vi "get_Jog.vi"(0 "路径":path, 2 "坐标转换":dbl[](array[numeric]), 3 "初始化？":bool, 4 "error in (no error)":errorcluster caption="错误输入（无错误）") -> (1 "上次限位":dbl, 5 "上一次位置":i32[](array[numeric]), 6 "File Out":path, 7 "坐标位置":dbl[][](array[numeric])=[[0.0, 1000.0, 2000.0, 3000.0], [0.0, 1000.0, 2000.0, 3000.0], [0.0, 1000.0, 2000.0, 3000.0], [0.0, 1000.0, 2000.0, 3000.0], [0.0, 1000.0, 2000.0, 3000.0]], 8 "当前位置":string[](array[string]), 9 "error out":errorcluster, 10 "工位名称":cluster{"String":string, "数值":i32}[](array[cluster]))   [LabVIEW 2018]
uses:
  <vilib>/Utility/file.llb/Write Delimited Spreadsheet (DBL).vi
  <vilib>/Utility/file.llb/Write Delimited Spreadsheet (string).vi
  <vilib>/Utility/file.llb/Read Delimited Spreadsheet (string).vi
panel:
  in  "table 4":string
  in  "table 3":string
  in  "table 2":string
  in  "table1":string
  in  "退出":bool caption="按钮"
  in  "确定":bool caption="按钮"
  in  "位置":dbl[][](array[numeric])=[[0.0, 100.0, 200.0, 300.0], [0.0, 100.0, 200.0, 300.0], [0.0, 100.0, 200.0, 300.0], [0.0, 1000.0, 2000.0, 3000.0], [0.0, 1000.0, 2000.0, 3000.0], [0.0, 1000.0, 2000.0, 3000.0]] min=0.0
  # "大平台X mm"
  # "大平台Y mm"
  # "大平台Z mm"
  # "小平台X mm"
  # "大平台Y mm"
  # "小平台Z mm"
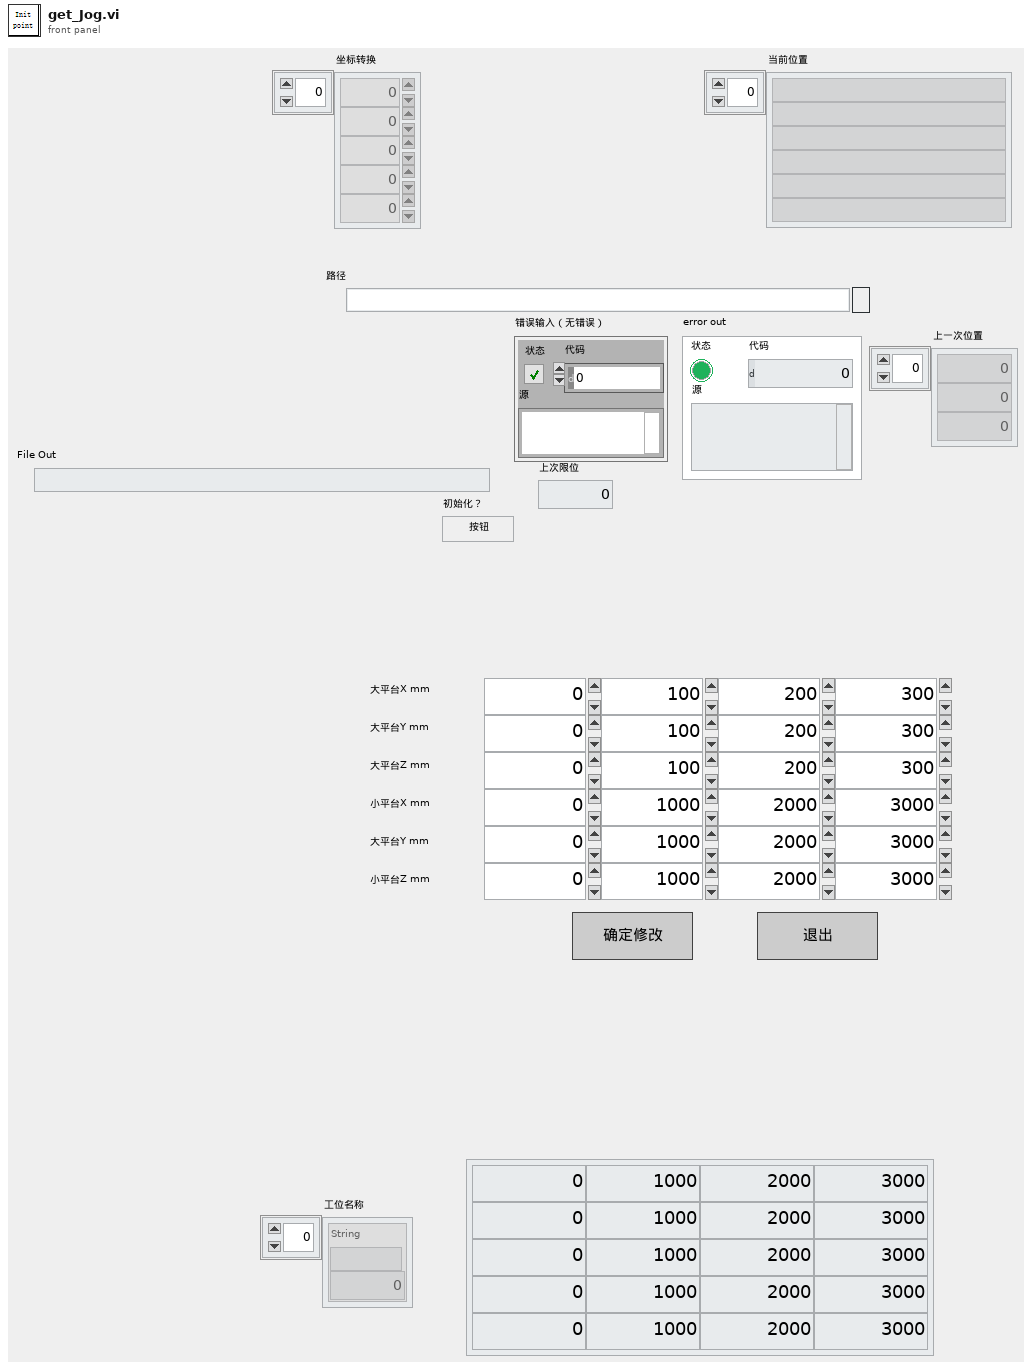
[diagram p1: front panel]
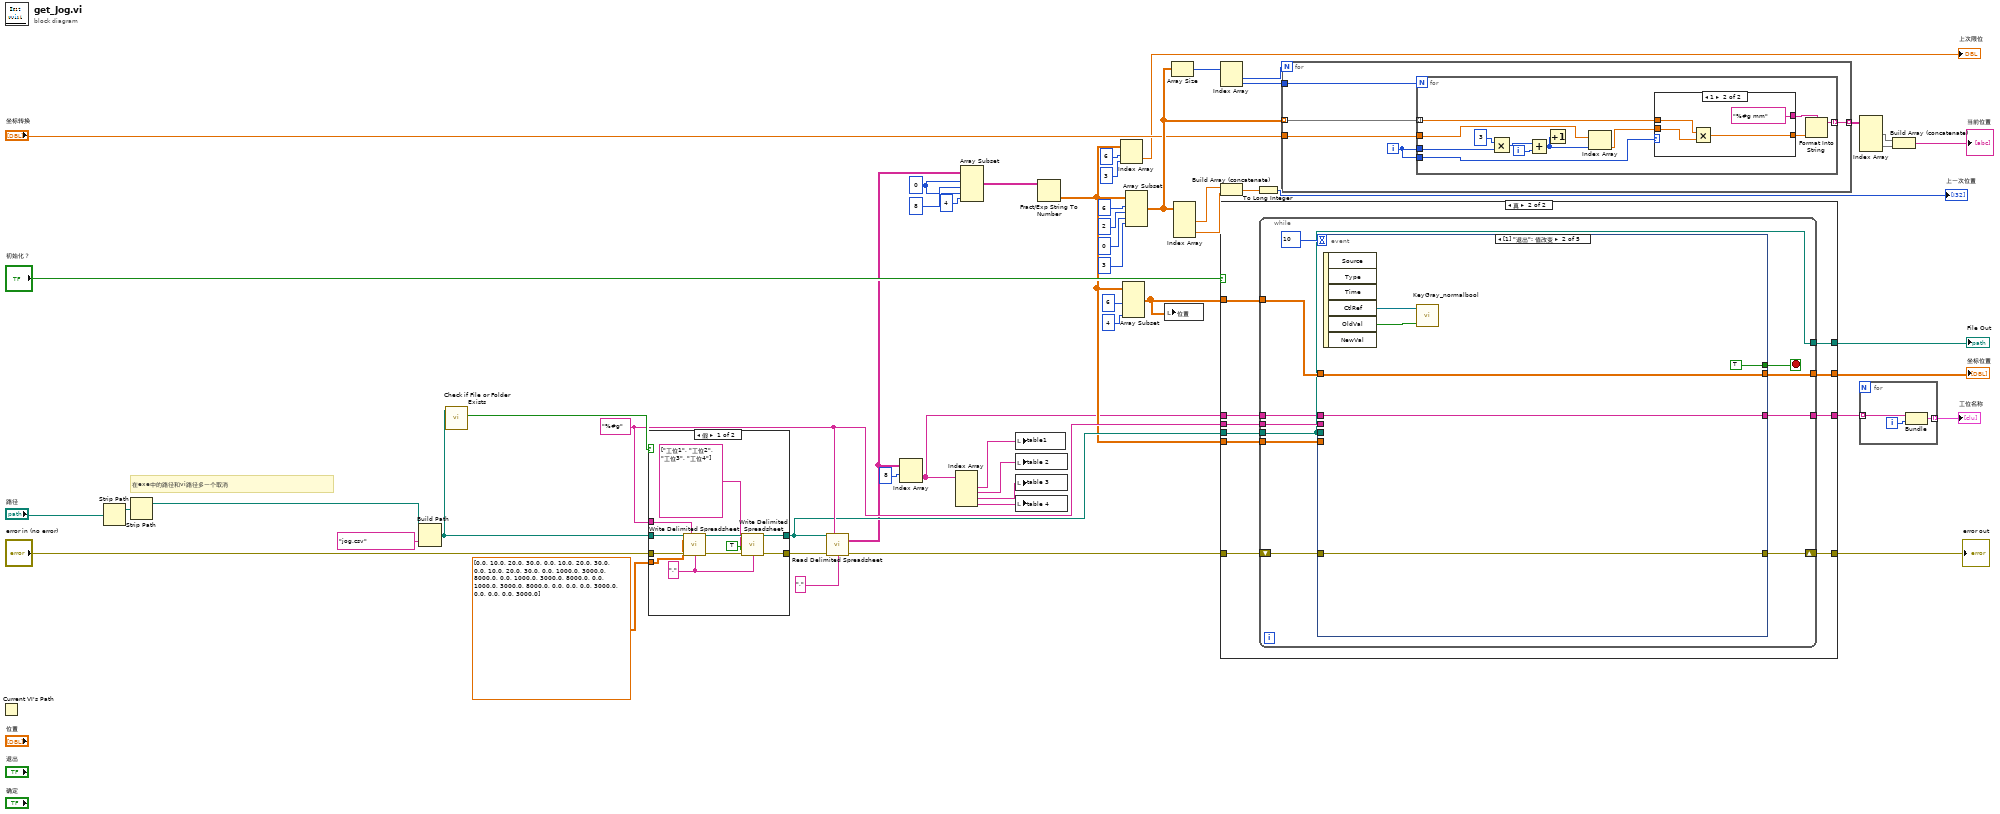
[diagram p0: block diagram]
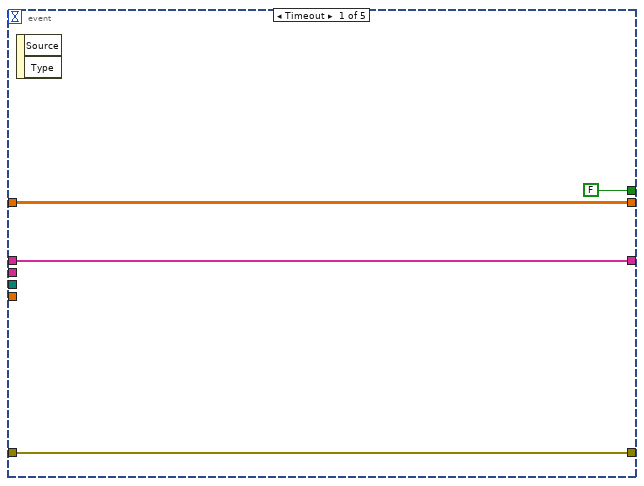
[diagram p3: hidden frame]
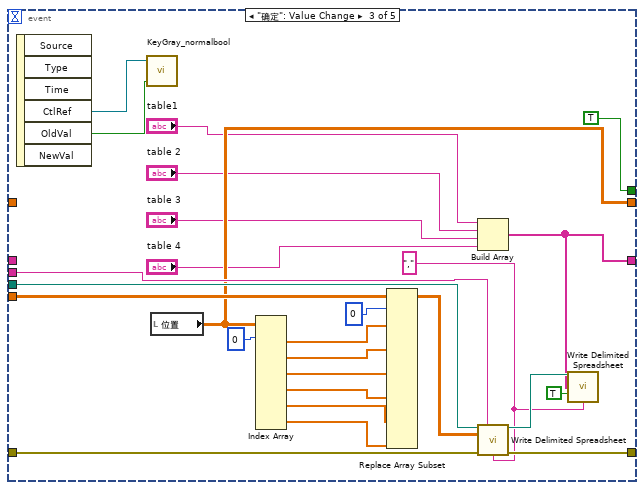
[diagram p4: hidden frame]
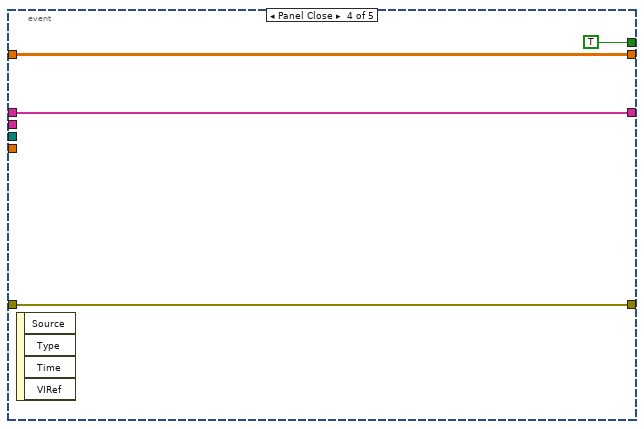
[diagram p5: hidden frame]
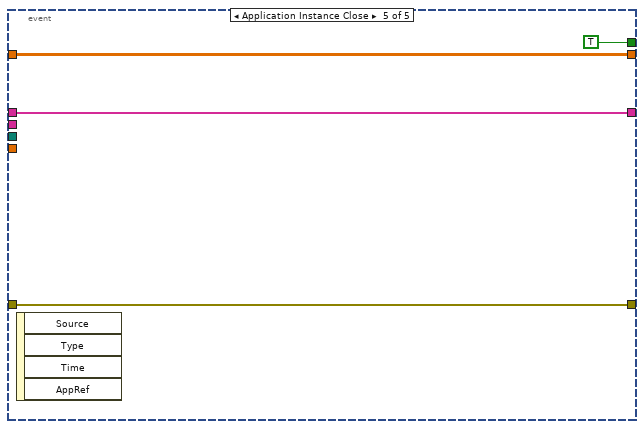
[diagram p6: hidden frame]
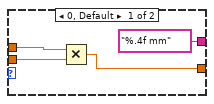
[diagram p7: hidden frame]
diagram:
  w13 = 0 ("索引")
  w47 = "%#g" ("format (%.3f)")
  # "在exe中的路径和vi路径多一个取消"
  n1 = Current VI's Path() -> ()  [unwired: 1 out]
  n2 = Strip Path(path="路径") -> (stripped path=w17:path)  [unwired: 1 out]
  n3 = Strip Path(path=w17) -> (stripped path=w16:path)  [unwired: 1 out]
  n4 = Build Path(base path=w16, name or relative path="jog.csv" ("名称或相对路径")) -> (appended path=w52:path)
  n5 = call <vilib>:"Check if File or Folder Exists.vi"("path"=w52) -> ("file or folder exists?"=w53:bool)  [unwired: 8 in, 2 out]
  n6 = case shown="假" w53 {
    tunnel: w52 -> [w65 w67]
    tunnel: [w59 w67] -> w37
    tunnel: w47 -> [w64 _]
    tunnel: "error in (no error)" -> [w63 w66]
    tunnel: [w58 w66] -> w50
    tunnel: dbl[][] [[0.0, 10.0, 20.0, 30.0], [0.0, 10.0, 20.0, 30.0], [0.0, 10.0, 20.0, 30.0], [0.0, 1000.0, 3000.0, 8000.0], [0.0, 1000.0, 3000.0, 8000.0], [0.0, 1000.0, 3000.0, 8000.0], [0.0, 0.0, 0.0, 3000.0], [0.0, 0.0, 0.0, 3000.0]] ("位置") -> [w62 _]
    frame False {
      w56 = "," ("delimiter (\\t)")
      n7 = call-poly <vilib>:"Write Delimited Spreadsheet.vi"("file path (dialog if empty)"=w65, "format (%.3f)"=w64, "2D data"=w62, "error in (no error)"=w63, "delimiter (\\t)"=w56) -> ("new file path (Not A Path if cancelled)"=w61:path, "error out"=w60:errorcluster)  [unwired: 9 in]
      n8 = call-poly <vilib>:"Write Delimited Spreadsheet.vi"("file path (dialog if empty)"=w61, "1D data"=string[] ["工位1", "工位2", "工位3", "工位4"], "append to file? (new file:F)"=TRUE, "error in (no error)"=w60, "delimiter (\\t)"=w56) -> ("new file path (Not A Path if cancelled)"=w59:path, "error out"=w58:errorcluster)  [unwired: 9 in]
    }
    frame True {
    }
  }
  n9 = call-poly <vilib>:"Read Delimited Spreadsheet.vi"("file path (dialog if empty)"=w37, "format (%s)"=w47, "error in (no error)"=w50, "delimiter (\\t)"="," ("delimiter (\\t)")) -> ("all rows"=w9:string[][], "error out"=w48:errorcluster)  [unwired: 6 in, 4 out]
  n10 = Index Array(array=w9, index (row)=8 ("索引 (行)")) -> (element=w1:string[])  [unwired: 1 in]
  n11 = Index Array(array=w1) -> (element #1=w6:string, element #2=w5:string, element #3=w4:string, element #4=w3:string)  [unwired: 4 in]
  n12 = Array Subset(array=w9, index (row)=w13, length (row)=8 ("长度"), index (col)=w13, length (col)=4 ("长度")) -> (w11:string[][])
  n13 = local write "table1"(w6) -> ()
  n14 = local write "table 2"(w5) -> ()
  n15 = local write "table 3"(w4) -> ()
  n16 = local write "table 4"(w3) -> ()
  n17 = Fract/Exp String To Number(string=w11) -> (number=w10:dbl[][])  [unwired: 3 in, 1 out]
  n18 = Index Array(array=w10, index (row)=6 ("索引 (行)"), index (col)=3 ("禁用的索引 (列)")) -> (element=→"上次限位":dbl)
  n19 = Array Subset(array=w10, length (row)=6 ("长度"), length (col)=4 ("长度")) -> (w42:dbl[][])  [unwired: 2 in]
  n20 = Array Subset(array=w10, index (row)=6 ("索引"), length (row)=2 ("长度"), index (col)=0 ("索引"), length (col)=3 ("长度")) -> (w28:dbl[][])
  n21 = local write "位置"(w42) -> ()
  n22 = Array Size(array=w28) -> (size(s)=w27:i32[])
  n23 = Index Array(array=w28) -> (element #1=w30:dbl[], element #2=w29:dbl[])  [unwired: 4 in]
  n24 = Index Array(array=w27) -> (element #1=w26:i32, element #2=w25:i32)  [unwired: 2 in]
  n25 = Build Array (concatenate)(w30, w29) -> (w23:dbl[])
  n26 = case shown="真" "初始化？" {
    tunnel: w48 -> [w69 w81]
    tunnel: w47 -> [_ w80]
    tunnel: [w69 w79] -> w46
    tunnel: [w70 w78] -> w45
    tunnel: w42 -> [w70 w77]
    tunnel: w37 -> [w71 w76]
    tunnel: [w71 w75] -> w31
    tunnel: w10 -> [_ w74]
    tunnel: [w68 w73] -> w2
    tunnel: w1 -> [w68 w72]
    frame False {
    }
    frame True {
      n27 = while {
        tunnel: w76 -> [w85]
        shift-right: [w90] -> w79
        shift-left: w81 -> [w91]
        tunnel: w80 -> [w89]
        tunnel: [w87] -> w78
        tunnel: w77 -> [w86]
        tunnel: [w85] -> w75
        tunnel: w74 -> [w84]
        tunnel: [w83] -> w73
        tunnel: w72 -> [w82]
        stop <- w88 stop-if-true
        n28 = event shown="[1] \"退出\": 值改变" {
          selector: _ -> [_ _ _ _ _]
          dyn-events: _ -> [_ _ _ _ _]
          timeout: 10 -> [_ _ _ _ _]
          tunnel: w85 -> [_ _ w128 _ _]
          tunnel: w91 -> [w95 w101 w127 w131 w135]
          tunnel: [w95 w101 w126 w131 w135] -> w90
          tunnel: w89 -> [_ _ w125 _ _]
          tunnel: [FALSE TRUE TRUE TRUE TRUE] -> w88
          tunnel: [w94 w100 w118 w130 w134] -> w87
          tunnel: w86 -> [w94 w100 _ w130 w134]
          tunnel: w84 -> [_ _ w120 _ _]
          tunnel: [w93 w97 w103 w129 w133] -> w83
          tunnel: w82 -> [w93 w97 _ w129 w133]
          event Timeout {
            n29 = event-data() -> ()  [unwired: 1 in, 2 out]
          }
          event "退出": Value Change {
            n30 = event-data() -> ("CtlRef"=w99:refnum<vi>, "OldVal"=w98:bool)  [unwired: 1 in, 4 out]
            n31 = call "KeyGray_normalbool.vi"("OldVal"=w98, "引用"=w99) -> ()  [unwired: 2 in]
          }
          event "确定": Value Change {
            w121 = "," ("delimiter (\\t)")
            n32 = event-data() -> ("CtlRef"=w109:refnum<vi>, "OldVal"=w108:bool)  [unwired: 1 in, 4 out]
            n33 = call "KeyGray_normalbool.vi"("OldVal"=w108, "引用"=w109) -> ()  [unwired: 2 in]
            n34 = local read "位置"() -> (w118:dbl[][])
            n35 = Index Array(array=w118, index (row) #1=0 ("索引 (行)")) -> (element #1=w116:dbl[], element #2=w115:dbl[], element #3=w114:dbl[], element #4=w113:dbl[], element #5=w112:dbl[], element #6=w111:dbl[])  [unwired: 11 in]
            n36 = Replace Array Subset(array=w120, new element #1=w116, index (row) #1=0 ("索引 (行)"), new element #2=w115, new element #3=w114, new element #4=w113, new element #5=w112, new element #6=w111) -> (w110:dbl[][])  [unwired: 11 in]
            n37 = Build Array("table1", "table 2", "table 3", "table 4") -> (w103:string[])
            n38 = call-poly <vilib>:"Write Delimited Spreadsheet.vi"("file path (dialog if empty)"=w128, "format (%.3f)"=w125, "2D data"=w110, "error in (no error)"=w127, "delimiter (\\t)"=w121) -> ("new file path (Not A Path if cancelled)"=w123:path, "error out"=w126:errorcluster)  [unwired: 9 in]
            n39 = call-poly <vilib>:"Write Delimited Spreadsheet.vi"("file path (dialog if empty)"=w123, "1D data"=w103, "append to file? (new file:F)"=TRUE, "delimiter (\\t)"=w121) -> ()  [unwired: 10 in, 2 out]
          }
          event Panel Close {
            n40 = event-data() -> ()  [unwired: 1 in, 4 out]
          }
          event Application Instance Close {
            n41 = event-data() -> ()  [unwired: 1 in, 4 out]
          }
        }
      }
    }
  }
  "error out" <- w46
  "坐标位置" <- w45
  "File Out" <- w31
  n42 = To Long Integer(number=w23) -> (32bit integer=→"上一次位置":i32[])
  n43 = for {
    N: w26 -> [_]
    tunnel: w28 -> [w141] mode=indexing
    tunnel: [w139] -> w36 mode=indexing
    tunnel: w25 -> [w138]
    tunnel: "坐标转换" -> [w137]
    i -> [w140]
    n44 = for {
      N: w138 -> [_]
      tunnel: w141 -> [w146] mode=indexing
      tunnel: w140 -> [w153]
      tunnel: w140 -> [w150]
      tunnel: [w148] -> w139 mode=indexing
      tunnel: w137 -> [w147]
      i -> [w143]
      n45 = Multiply(x=3, y=w150) -> (x*y=w149:i32)
      n46 = Add(x=w149, y=w143) -> (x+y=w142:i32)
      n47 = Increment(x=w142) -> ()  [unwired: 1 out]
      n48 = Index Array(array=w147, index=w142) -> (element=w145:dbl)
      n49 = case shown="1" w153 {
        tunnel: ["%.4f mm" ("格式字符串") "%#g mm" ("格式字符串")] -> w152
        tunnel: w146 -> [w156 w160]
        tunnel: w145 -> [w155 w159]
        tunnel: [w154 w158] -> w144
        frame 0, Default {
          n50 = Multiply(x=w156, y=w155) -> (x*y=w154:dbl)
        }
        frame 1 {
          n51 = Multiply(x=w160, y=w159) -> (x*y=w158:dbl)
        }
      }
      n52 = Format Into String(format string=w152, w144) -> (resulting string=w148:string)  [unwired: 2 in, 1 out]
    }
  }
  n53 = Index Array(array=w36) -> (element #1=w35:string[], element #2=w34:string[])  [unwired: 4 in]
  n54 = for {
    tunnel: [w163] -> w7 mode=indexing
    tunnel: w2 -> [w162] mode=indexing
    i -> [w164]
    n55 = Bundle("String"=w162, w164) -> (w163:cluster{"String":string, i32})  [unwired: 1 in]
  }
  "工位名称" <- w7
  n56 = Build Array (concatenate)(w35, w34) -> (→"当前位置":string[])
